vi "IndoorMonitoring_Main.vi"() -> ()   [LabVIEW 2014]
uses:
  IndoorData_class/DebugData.ctl
  IndoorData_class/ActualValues.ctl
  <vilib>/Platform/TimedLoop/XDataNode/timing_clust.ctl
  <vilib>/Platform/TimedLoop/XDataNode/nitl_modes.ctl
  <vilib>/Platform/TimedLoop/XDataNode/wakeup.ctl
  <vilib>/MakerHub/LINX/Public/Peripherals/Digital/Digital Write 1 Chan.vi
  <vilib>/MakerHub/LINX/Public/Peripherals/Digital/Digital Write N Chans.vi
  <vilib>/MakerHub/LINX/Private/Local IO/LinxDigitalWrite.vi
  <vilib>/MakerHub/LINX/Public/Utilities/Check Channel.vi
  <vilib>/MakerHub/LINX/Private/Local IO/Handle Errors.vi
  <vilib>/MakerHub/LINX/Public/Utilities/Open Local.vi
  <vilib>/MakerHub/LINX/Private/Utilties/Generate Error.vi
  <vilib>/platform/TimedLoop/XDataNode/XDataNode.xnode
  Sensor_SHT21/SHT21_class/SHT21.lvclass
  IndoorData_class/IndoorData.lvclass
  <vilib>/Platform/TimedLoop/XDataNode/XDNodeRunTimeDep.lvlib
  <vilib>/MakerHub/LINX/LMH-LINX.lvlib
panel:
  out "ActualValues":T1
  out "DebugData":T2
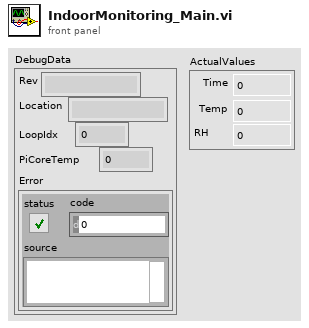
[diagram p1: front panel]
types:
  T1 = typedef "IndoorData.lvclass/ActualValues.ctl" = cluster{"Time":dbl, "Temp":dbl, "RH":dbl}
  T2 = typedef "IndoorData.lvclass/DebugData.ctl" = cluster{"Rev":string, "Location":string, "LoopIdx":i32, "PiCoreTemp":dbl, "Error":errorcluster}
  T3 = typedef "LMH-LINX.lvlib/LINX Ref.ctl" = cluster{"IO":T4, "Interface":T5, "LINX Device Config":T6}
  T4 = typedef "LMH-LINX.lvlib/Platform.ctl" = enum16{"Remote", "Local"}
  T5 = typedef "LMH-LINX.lvlib/Interface.ctl" = enum16{"Serial", "TCP"}
  T6 = typedef "LMH-LINX.lvlib/Device.lvlib/LINX Device Config.ctl" = cluster{"Interface":T5, "COM Port":refnum<visa-resource-name>, "TCP Configuration":T7, "Device Family":u8, "Device ID":u8, "Device Name":string, "TCP Ref":refnum<k5>, "Channels":T8}
  T7 = typedef "LMH-LINX.lvlib/Device.lvlib/TCP Config.ctl" = cluster{"IP Address":string, "Port":u16}
  T8 = typedef "LMH-LINX.lvlib/Channels.ctl" = cluster{"DI":u8[], "DO":u8[], "AI":u8[], "AO":u8[], "PWM":u8[], "QE":u8[], "UART":u8[], "I2C 2":u8[], "SPI":u8[], "CAN":u8[], "Servo":u8[], "AI Ref (V)":dbl, "AI Resolution (Bits)":u8, "AO Ref (V)":dbl, "AO Resolution (Bits)":u8}
  T9 = typedef "XDNodeRunTimeDep.lvlib/timing_clust.ctl" = cluster{"Expected End [f-1]":u64, "Actual End [f-1]":u64, "Finished Late? [f-1]":bool, "Expected End [i-1]":u64, "Actual End [i-1]":u64, "Finished Late? [i-1]":bool, "Expected Start [i]":u64, "Actual Start [i]":u64, "Expected Start [f]":u64, "Actual Start [f]":u64, "Source Name":string, "Structure Name":string, "Period":i64, "Deadline":i64, "Offset":i64, "Start":i64, "Priority":i32, "Timeout":i32, "Mode":T10, "Wakeup Reason":T11, "Error":errorcluster, "Source Type":string, "Secondary Source Type":string, "Global End Time":u64, "Global Start Time":u64, "Frame Duration":u64, "Iteration Duration":u64, "Assigned CPU":i32, "I/O Scan Engine Mode":u32}
  T10 = typedef "XDNodeRunTimeDep.lvlib/nitl_modes.ctl" = enum32{"No Change", "Process missed periods, maintain original phase", "Discard missed periods, maintain original phase", "Process missed periods, ignore original phase", "Discard missed periods, ignore original phase"}
  T11 = typedef "XDNodeRunTimeDep.lvlib/wakeup.ctl" = enum32{"Normal", "Aborted", "Asynchronous wakeup", "Timing source error", "Timed loop error", "Timeout"}
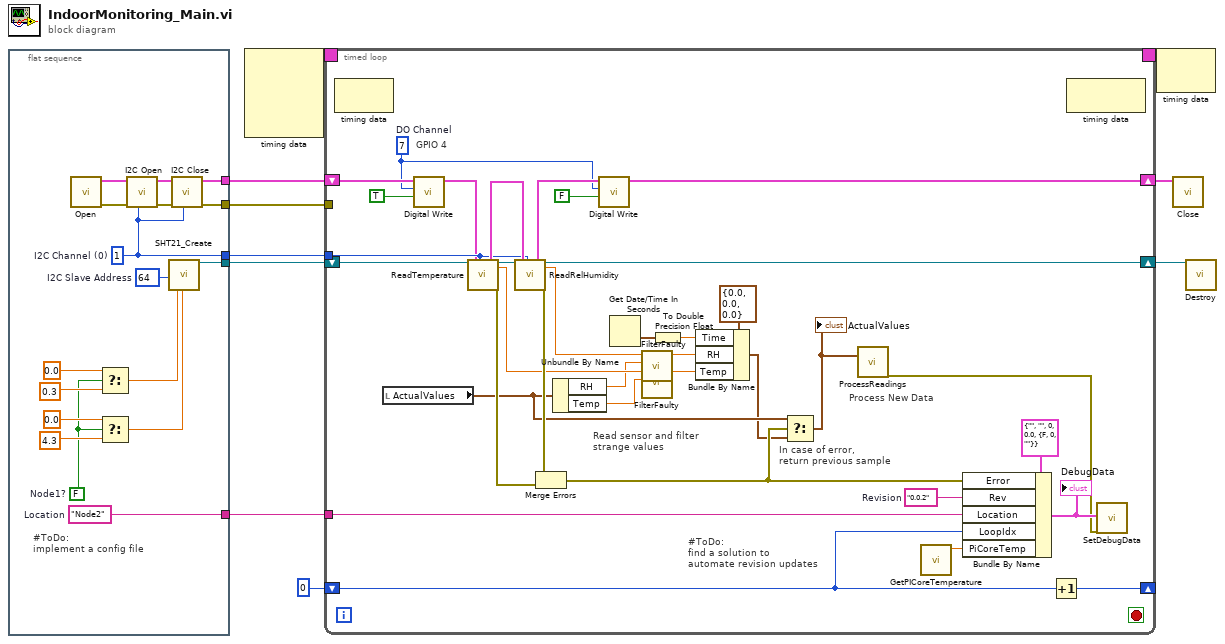
[diagram p0: block diagram]
diagram:
  n1 = flat-sequence {
    tunnel: [w23] -> w7
    tunnel: [w22] -> w6
    tunnel: [w21] -> w4
    tunnel: [w19] -> w2
    tunnel: [w18] -> w1
    frame #0 {
      w11 = FALSE  # Node1?
      w18 = "Node2"  # Location
      w20 = u8 64  # I2C Slave Address
      w19 = u8 1  # I2C Channel (0)
      # "#ToDo:\nimplement a config file"
      n2 = call-poly <vilib>:"Open.vi"() -> ("Error Out"=w25:errorcluster, "LINX Resource"=w27:T3)  [unwired: 9 in, 1 out]
      n3 = Select(t=0.0, s=w11, f=0.3 ("t")) -> (s? t:f=w15:dbl)
      n4 = Select(t=0.0, s=w11, f=4.3 ("t")) -> (s? t:f=w12:dbl)
      n5 = call <vilib>:"I2C Open.vi"("I2C Channel (0)"=w19, "Error In"=w25, "LINX Resource"=w27) -> ("Error Out"=w24:errorcluster, "LINX Resource"=w26:T3)  [unwired: 7 in]
      n6 = call "SHT21_Create.vi"("I2C Slave Address (0)"=w20, "T Offset"=w15, "RH Offset"=w12) -> ("reference out"=w21:refnum<class "SHT21.lvclass">)  [unwired: 15 in, 1 out]
      n7 = call <vilib>:"I2C Close.vi"("I2C Channel (0)"=w19, "Error In"=w24, "LINX Resource"=w26) -> ("Error Out"=w22:errorcluster, "LINX Resource"=w23:T3)  [unwired: 7 in]
    }
  }
  n8 = node-c288() -> (w10:T9)  [unwired: 4 in]
  n9 = timed-loop {
    timing: w10 -> [_]
    timing-out: [_] -> w9
    shift-right: [w59] -> _
    shift-left: 0 -> [w39]
    shift-right: [w43] -> w5
    shift-left: w7 -> [w47]
    tunnel: w6 -> [_]
    shift-right: [w55] -> w3
    shift-left: w4 -> [w57]
    tunnel: w2 -> [w53]
    tunnel: w1 -> [w41]
    stop <- _ stop-if-true
    w28 = u8 7  # DO Channel
    w58 = "0.0.2"  # Revision
    # "#ToDo:\nfind a solution to\nautomate revision updates"
    # "Process New Data"
    # "Read sensor and filter\nstrange values"
    # "In case of error,\nreturn previous sample"
    # "GPIO 4"
    n10 = node-c288() -> ()  [unwired: 1 in, 1 out]
    n11 = local read "ActualValues"() -> (w31:T1)
    n12 = call-poly <vilib>:"Digital Write.vi"("Output Value"=TRUE, "DO Channel"=w28, "LINX Resource"=w47) -> ("LINX Resource"=w46:T3)  [unwired: 7 in, 1 out]
    n13 = call-dynamic "ReadTemperature.vi"("reference in"=w57, "LINX Resource"=w46, "I2C Channel (0)"=w53) -> ("LINX Resource"=w54:T3, "reference out"=w56:refnum<class "SHT21.lvclass">, "Temperature"=w35:dbl, "error out"=w52:errorcluster)  [unwired: 12 in, 1 out]
    n14 = call-dynamic "ReadRelHumidity.vi"("reference in"=w56, "LINX Resource"=w54, "I2C Channel (0)"=w53) -> ("LINX Resource"=w44:T3, "reference out"=w55:refnum<class "SHT21.lvclass">, "RH"=w38:dbl, "error out"=w51:errorcluster)  [unwired: 12 in, 1 out]
    n15 = Merge Errors(w51, w52) -> (w32:errorcluster)
    n16 = Unbundle By Name(w31) -> ("RH"=w34:dbl, "Temp"=w33:dbl)
    n17 = call-poly <vilib>:"Digital Write.vi"("Output Value"=FALSE, "DO Channel"=w28, "LINX Resource"=w44) -> ("LINX Resource"=w43:T3)  [unwired: 7 in, 1 out]
    n18 = Get Date/Time In Seconds() -> (seconds since 1Jan1904=w48:timestamp)
    n19 = call "FilterFaulty.vi"("Prev. Measurement In"=w34, "Measurement In"=w38) -> ("Measurement Out"=w37:dbl)  [unwired: 9 in]
    n20 = call "FilterFaulty.vi"("Prev. Measurement In"=w33, "Measurement In"=w35) -> ("Measurement Out"=w36:dbl)  [unwired: 9 in]
    n21 = To Double Precision Float(number=w48) -> (double precision float=w49:dbl)
    n22 = Bundle By Name(cluster=T1 {"Time"=0.0, "Temp"=0.0, "RH"=0.0} ("ActualValues"), "Time"=w49, "RH"=w37, "Temp"=w36) -> (w30:T1)
    n23 = Select(t=w31, s=w32, f=w30) -> (s? t:f=w29:T1)
    "ActualValues" <- w29
    n24 = call "ProcessReadings.vi"("ActualValues"=w29) -> ("error out"=w40:errorcluster)  [unwired: 18 in]
    n25 = call "GetPICoreTemperature.vi"() -> ("PICoreTemp"=w62:dbl)  [unwired: 10 in, 1 out]
    n26 = Bundle By Name(cluster=T2 {"Rev"="", "Location"="", "LoopIdx"=0, "PiCoreTemp"=0.0, "Error"={"status"=FALSE, "code"=0, "source"=""}} ("DebugData"), "Error"=w32, "Rev"=w58, "Location"=w41, "LoopIdx"=w39, "PiCoreTemp"=w62) -> (w61:T2)
    "DebugData" <- w61
    n27 = Increment(x=w39) -> (x+1=w59:i32)
    n28 = node-c288() -> ()  [unwired: 1 in, 1 out]
    n29 = call "SetDebugData.vi"("DebugData"=w61, "error in (no error)"=w40) -> ()  [unwired: 17 in, 1 out]
  }
  n30 = node-c288(w9) -> ()  [unwired: 1 out]
  n31 = call <vilib>:"Close.vi"("LINX Resource"=w5) -> ()  [unwired: 10 in, 1 out]
  n32 = call-dynamic "Destroy.vi"("reference in"=w3) -> ()  [unwired: 17 in, 2 out]
